vi "Test - With DRAM.vi"() -> ()   [LabVIEW 2020, in "Raster (FPGA).lvlib"]
uses:
  Raster (FPGA).lvlib
  Triangle.ctl
  Vertex.ctl
  Vector 3D.ctl
  UV.ctl
  <vilib>/rvi/Emulation/niFpgaGetClockAttributes.vi
  <vilib>/rvi/Emulation/niFpgaSctlEmulationGetInTimedLoop.vi
  <vilib>/rvi/Emulation/niFpgaEmulationReportErrorSimple.vi
  <vilib>/rvi/Emulation/niFpgaCriticalErrorInLSC.vi
  <vilib>/rvi/DataTransferAndStorage/Container/XNode/niFpgaContainer.xnode
  <vilib>/rvi/Memory/Memory_Emulation/niFpgaMemoryFastEmulationDramWriteAndRequestData.vi
  <vilib>/rvi/Memory/Memory_Emulation/niFpgaMemoryEmulationDramWriteAndRequestData.vi
  <vilib>/platform/TimedLoop/XDataNode/XDataNode.xnode
  <vilib>/Platform/TimedLoop/XDataNode/nitl_modes.ctl
  <vilib>/Platform/TimedLoop/XDataNode/XDNodeRunTimeDep.lvlib
  <vilib>/Platform/TimedLoop/XDataNode/wakeup.ctl
  <vilib>/Platform/TimedLoop/XDataNode/timing_clust.ctl
  <vilib>/rvi/interface/RandomDataEmulation/nirviRandomDataFpgaReadWriteTemplate.vi
  <vilib>/rvi/FIFO/Fifo_Resource/nirvififoEmulationRead.vi
  <vilib>/rvi/FIFO/Fifo_Resource/nirvififoEmulationWrite.vi
  <instrlib>/_niInstr/Basic Elements/v1/FPGA/niInstr Basic Elements v1 FPGA.lvlib
  <vilib>/rvi/Memory/Memory_Emulation/niFpgaMemoryEmulationDramRetrieveData.vi
panel:
  out "Element":cluster{"Address":i32, "Value":u32}
  out "To Host Timed Out? 2":bool
  in  "Send To Host 2":bool
  out "DRAM Read Address 2":u32
  out "Raster Loop Period [us]":u32
  in  "Raster Loop Wait [ticks]":u32=10000 caption="Count(uSec)"
  out "To DRAM Timed Out?":bool
  out "Raster Loop Index":i32
  in  "Triangle":T1={"Vertex 1"={"Position"={"x"=75.0, "y"=25.0, "z"=0.0}, "UV"={"u"=0.0, "v"=0.0}, "Colour"=12517256}, "Vertex 2"={"Position"={"x"=500.0, "y"=450.0, "z"=0.0}, "UV"={"u"=0.0, "v"=0.0}, "Colour"=12517256}, "Vertex 3"={"Position"={"x"=50.0, "y"=200.0, "z"=0.0}, "UV"={"u"=0.0, "v"=0.0}, "Colour"=12517256}, "Colour"=5308226} {"Vertex 3"."UV"."v" min=0 max=1 step=0.1; "Vertex 3"."UV"."u" min=0 max=1 step=0.1; "Vertex 2"."UV"."v" min=0 max=1 step=0.1; "Vertex 2"."UV"."u" min=0 max=1 step=0.1; "Vertex 1"."UV"."v" min=0 max=1 step=0.1; "Vertex 1"."UV"."u" min=0 max=1 step=0.1}
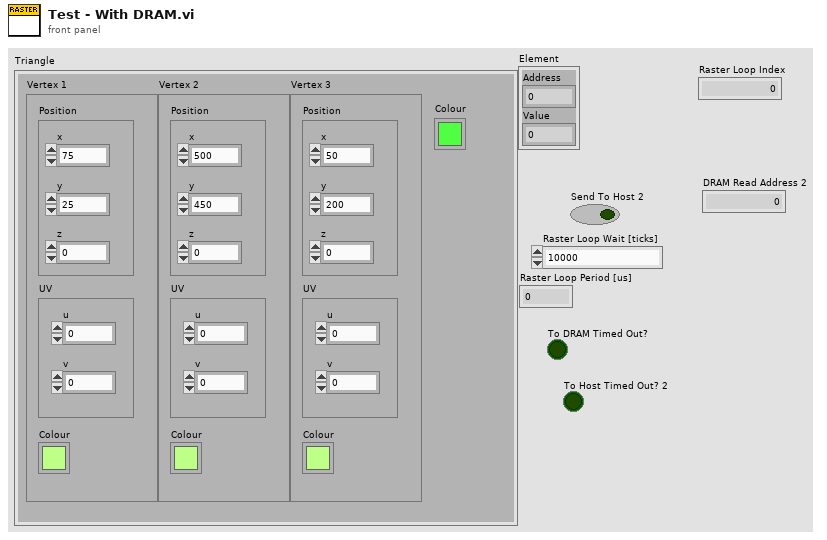
[diagram p1: front panel]
types:
  T1 = typedef "Raster (FPGA).lvlib/Triangle.ctl" = cluster{"Vertex 1":T2, "Vertex 2":T2, "Vertex 3":T2, "Colour":u32}
  T2 = typedef "Raster (FPGA).lvlib/Vertex.ctl" = cluster{"Position":T3, "UV":T4, "Colour":u32}
  T3 = typedef "Raster (FPGA).lvlib/Vector 3D.ctl" = cluster{"x":sgl, "y":sgl, "z":sgl}
  T4 = typedef "Raster (FPGA).lvlib/UV.ctl" = cluster{"u":sgl, "v":sgl}
  T5 = typedef "Raster (FPGA).lvlib/Triangle (Sorted).ctl" = cluster{"Top Vertex":T2, "Mid Vertex":T2, "Bottom Vertex":T2, "Colour":u32}
  T6 = typedef "Raster (FPGA).lvlib/Reciprocals.ctl" = cluster{"Bottom --> Top":sgl, "Bottom --> Middle":sgl, "Middle --> Top":sgl}
  T7 = typedef "Raster (FPGA).lvlib/Current Row.ctl" = cluster{"Start Column":sgl, "End Column":sgl}
  T8 = typedef "XDNodeRunTimeDep.lvlib/timing_clust.ctl" = cluster{"Expected End [f-1]":u64, "Actual End [f-1]":u64, "Finished Late? [f-1]":bool, "Expected End [i-1]":u64, "Actual End [i-1]":u64, "Finished Late? [i-1]":bool, "Expected Start [i]":u64, "Actual Start [i]":u64, "Expected Start [f]":u64, "Actual Start [f]":u64, "Source Name":string, "Structure Name":string, "Period":i64, "Deadline":i64, "Offset":i64, "Start":i64, "Priority":i32, "Timeout":i32, "Mode":T9, "Wakeup Reason":T10, "Error":errorcluster, "Source Type":string, "Secondary Source Type":string, "Global End Time":u64, "Global Start Time":u64, "Frame Duration":u64, "Iteration Duration":u64, "Assigned CPU":i32, "I/O Scan Engine Mode":u32}
  T9 = typedef "XDNodeRunTimeDep.lvlib/nitl_modes.ctl" = enum32{"No Change", "Process missed periods, maintain original phase", "Discard missed periods, maintain original phase", "Process missed periods, ignore original phase", "Discard missed periods, ignore original phase"}
  T10 = typedef "XDNodeRunTimeDep.lvlib/wakeup.ctl" = enum32{"Normal", "Aborted", "Asynchronous wakeup", "Timing source error", "Timed loop error", "Timeout"}
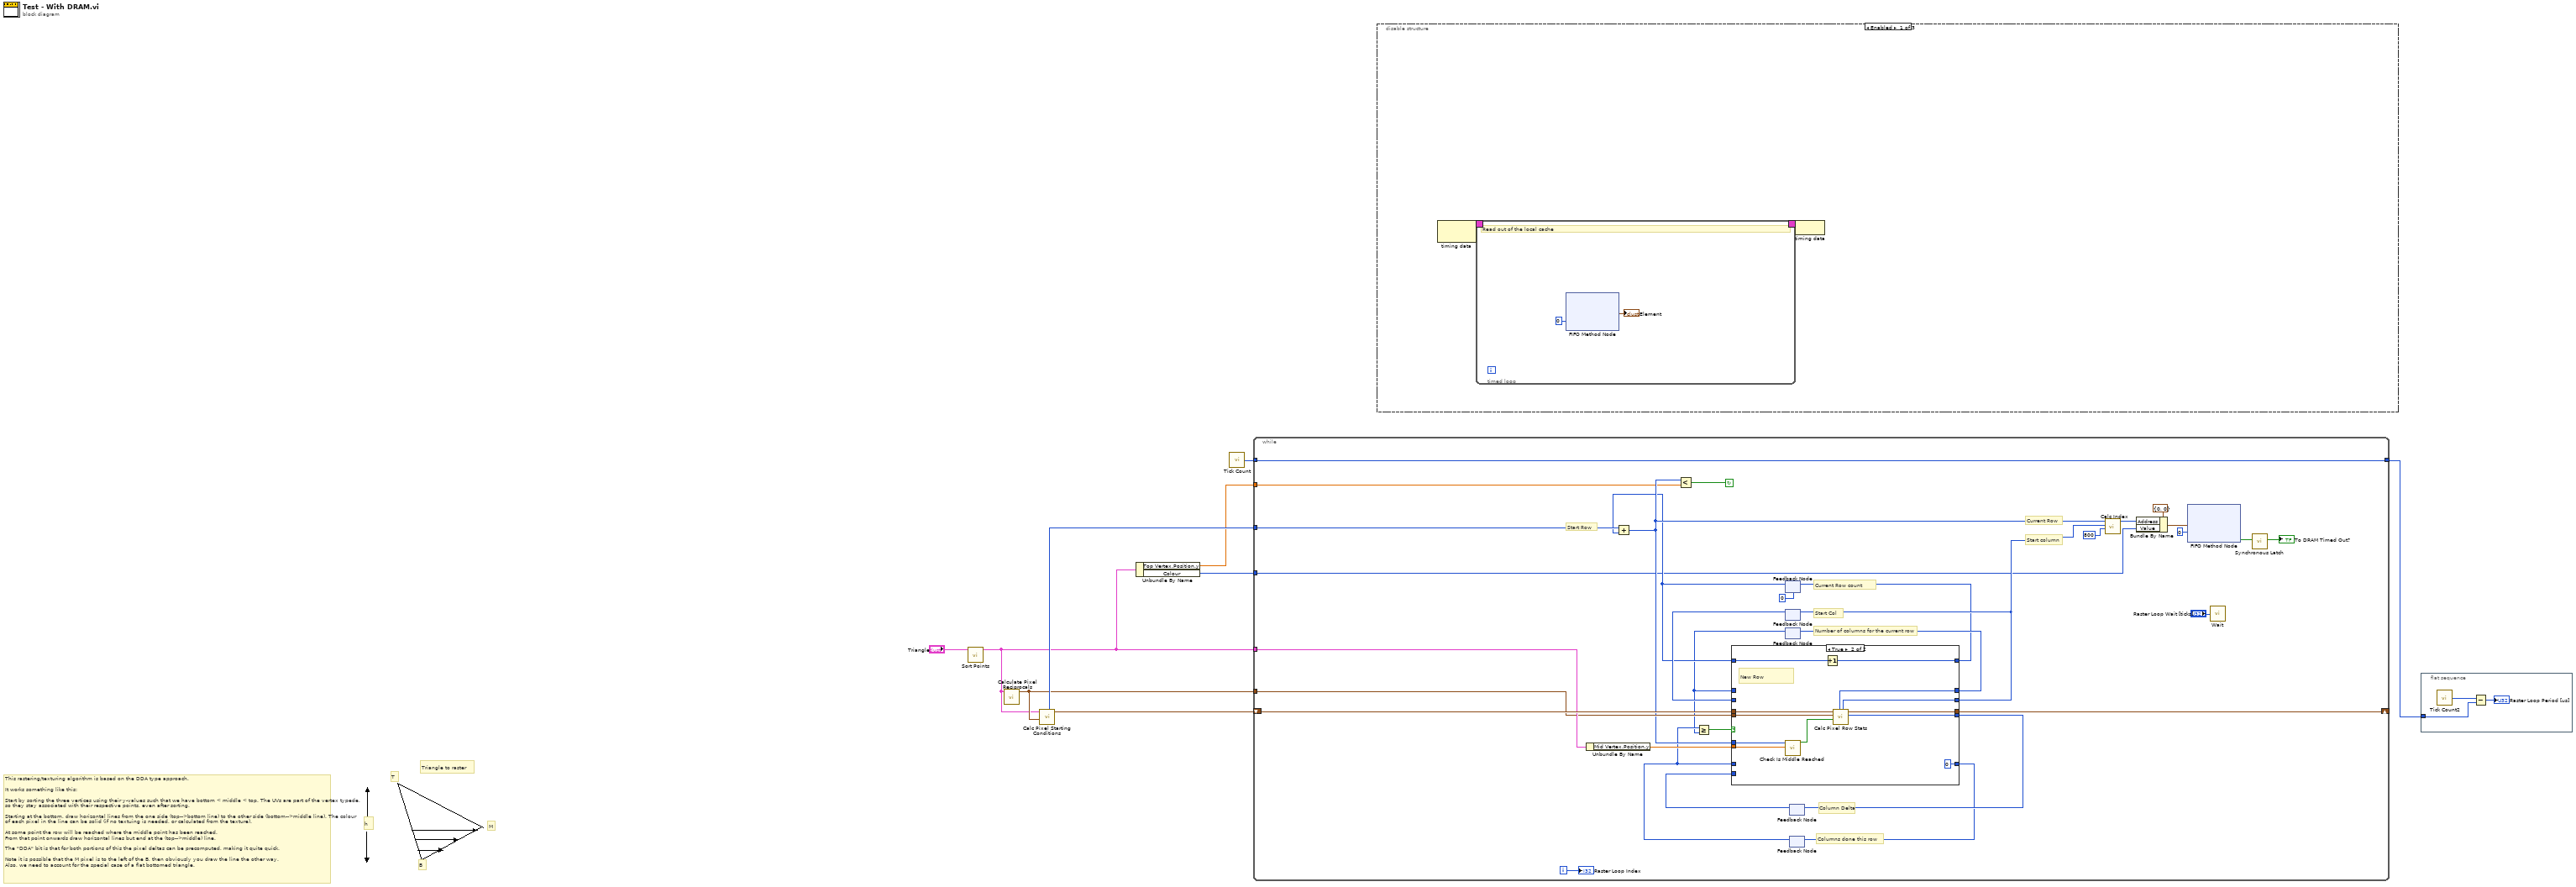
[diagram p0: block diagram]
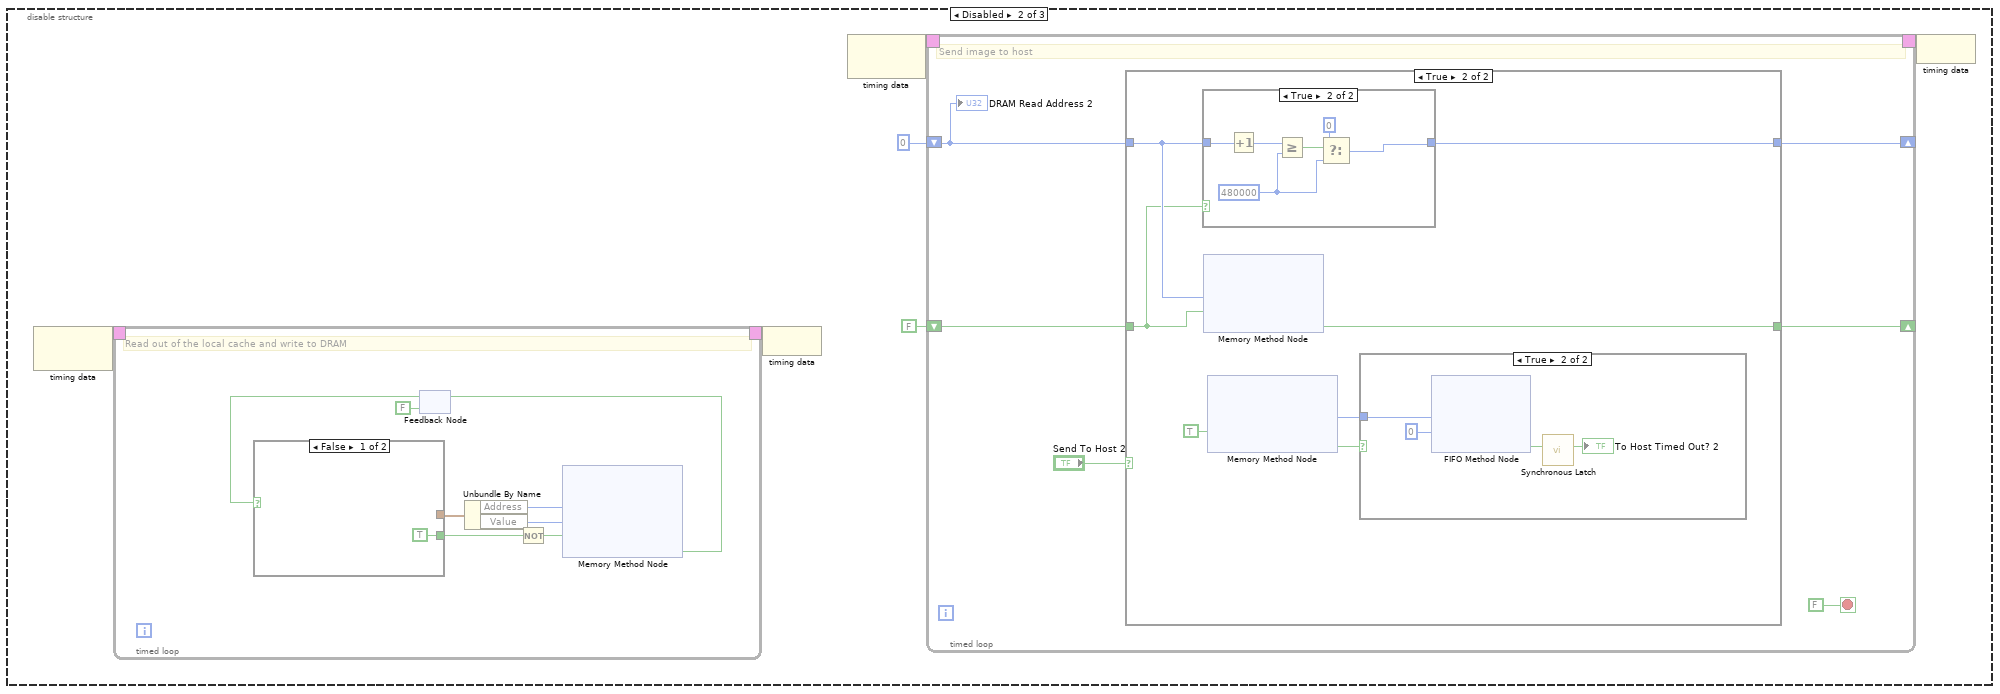
[diagram p2: hidden frame]
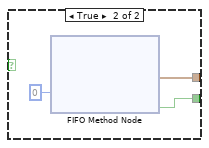
[diagram p6: hidden frame]
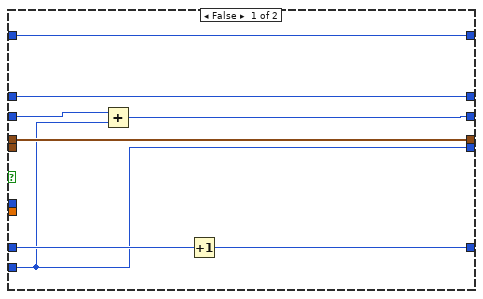
[diagram p8: hidden frame]
diagram:
  # "h"
  # "Triangle to raster"
  # "M"
  # "T"
  # "B"
  # "This rastering/texturing algorithm is based on the DDA type approach.\n\nIt works something like this:\n\nStart by sorting the three vertices using their y-values such that we have bottom < middle < top. The UVs are part of the vertex typede, so they stay associated with their respective points, even after sorting.\n\nStarting at the bottom, draw horizontal lines from the one side (top-->bottom line) to the other side (bottom-->middle line). The colour of each pixel in the line can be solid (if no textuing is needed, or calculated from the texture).\n\nAt some point the row will be reached where the middle point has been reached.\nFrom that point onwards draw horizontal lines but end at the (top-->middle) line.\n\nThe \"DDA\" bit is that for both portions of this the pixel deltas can be precomputed, making it quite quick.\n\nNote it is possible that the M pixel is to the left of the B, then obviously you draw the line the other way.\nAlso, we need to account for the special case of a flat bottomed triangle."
  n1 = call "Sort Points.vi"("Triangle"="Triangle") -> ("Sorted Triangle"=w4:T5)  [unwired: 10 in]
  n2 = call "Calculate Pixel Reciprocals.vi"("Sorted Triangle"=w4) -> ("Columns Pixels Per Row"=w6:T6)  [unwired: 10 in]
  n3 = call "Calc Pixel Starting Conditions.vi"("Reciprocals"=w6, "Sorted Vertices (V1 is top)"=w4) -> ("Start Row Columns"=w9:T7, "Start Row"=w8:i32)  [unwired: 8 in]
  n4 = Unbundle By Name(w4) -> ("Top Vertex.Position.y"=w3:sgl, "Colour"=w5:u32)
  n5 = call "Tick Count"() -> ("Tick Count(uSec)"=w2:u32)
  n6 = while {
    shift-right: [w39] -> _
    shift-left: w9 -> [w37]
    tunnel: w4 -> [w36]
    tunnel: w8 -> [w38]
    tunnel: w6 -> [w34]
    tunnel: w5 -> [w15]
    tunnel: w3 -> [w32]
    tunnel: w2 -> [w13]
    tunnel: [w13] -> w1
    i -> [w35]
    stop <- w40 continue-if-true
    # "Columns done this row"
    # "Column Delta"
    # "Current Row count"
    # "Start Col"
    # "Number of columns for the current row"
    # "Current Row"
    # "Start column"
    # "Start Row"
    n7 = Unbundle By Name(w36) -> ("Mid Vertex.Position.y"=w41:sgl)
    n8 = feedback #1(0) -> (w24:i32)
    n9 = Add(x=w38, y=w24) -> (x+y=w33:i32)
    n10 = Less?(x=w33, y=w32) -> (x < y?=w40:bool)
    n11 = feedback #2() -> (w29:i32)  [unwired: 1 in]
    n12 = feedback #3() -> (w21:i32)  [unwired: 1 in]
    n13 = feedback #4() -> (w27:i32)  [unwired: 1 in]
    n14 = feedback #5() -> (w22:i32)  [unwired: 1 in]
    n15 = Greater Or Equal?(x=w22, y=w21) -> (x >= y?=w20:bool)
    n16 = case shown="True" w20 {
      tunnel: w41 -> [_ w61]
      tunnel: [w48 w60] -> w39
      tunnel: w37 -> [w48 w59]
      tunnel: w34 -> [_ w58]
      tunnel: [w49 w57] -> w31
      tunnel: [w42 w55] -> w28
      tunnel: [w43 w54] -> w30
      tunnel: w33 -> [_ w53]
      tunnel: w21 -> [w49 _]
      tunnel: w29 -> [w44 _]
      tunnel: w27 -> [w42 _]
      tunnel: w24 -> [w47 w52]
      tunnel: [w47 w51] -> w25
      tunnel: [w45 0] -> w23
      tunnel: w22 -> [w46 _]
      frame False {
        n17 = Add(x=w44, y=w42) -> (x+y=w43:i32)
        n18 = Increment(x=w46) -> (x+1=w45:i32)
      }
      frame True {
        # "New Row"
        n19 = call "Check Is Middle Reached.vi"("Middle y"=w61, "Current Row"=w53) -> ("Reached Middle"=w56:bool)  [unwired: 9 in]
        n20 = Increment(x=w52) -> (x+1=w51:i32)
        n21 = call "Calc Pixel Row Stats.vi"("Reached Middle"=w56, "Reciprocals"=w58, "Current Row"=w59) -> ("Column Delta"=w55:i32, "Next Row"=w60:T7, "Start Col"=w54:i32, "Number Of Cols This Row"=w57:i32)  [unwired: 4 in, 1 out]
      }
    }
    n22 = feedback-in #1(w25) -> ()
    n23 = feedback-in #2(w30) -> ()
    n24 = feedback-in #3(w31) -> ()
    n25 = feedback-in #4(w28) -> ()
    n26 = feedback-in #5(w23) -> ()
    n27 = call "Calc Index.vi"("Cols Per Row"=800, "Col"=w30, "Row"=w33) -> ("Index"=w16:i32)  [unwired: 8 in]
    n28 = Bundle By Name(cluster=cluster{"Address":i32, "Value":u32} {"Address"=0, "Value"=0} ("Element"), "Address"=w16, "Value"=w15) -> (w17:cluster{"Address":i32, "Value":u32})
    n29 = xnode ("FIFO Method Node")("Element"=w17, "Timeout"=0) -> ("Timed Out?"=w10:bool)  [unwired: 1 in, 1 out]
    n30 = call "Wait"("Count(Ticks)"="Raster Loop Wait [ticks]") -> ()  [unwired: 1 out]
    n31 = call <instrlib>:"Synchronous Latch.vi"("set"=w10) -> ("out"=→"To DRAM Timed Out?":bool)  [unwired: 10 in]
    "Raster Loop Index" <- w35
  }
  n32 = disable-structure shown="Enabled" {
    frame Enabled {
      n33 = node-c288() -> (w63:T8)  [unwired: 1 in]
      n34 = timed-loop {
        timing: w63 -> [_]
        timing-out: [_] -> w62
        stop <- FALSE stop-if-true
        # "Read out of the local cache"
        n35 = xnode ("FIFO Method Node")("Timeout"=0) -> ("Element"=→"Element":cluster{"Address":i32, "Value":u32})  [unwired: 1 in, 2 out]
      }
      n36 = node-c288(w62) -> ()
    }
    frame Disabled {
      n37 = node-c288() -> (w76:T8)  [unwired: 1 in]
      n38 = timed-loop {
        timing: w76 -> [_]
        timing-out: [_] -> w75
        stop <- FALSE stop-if-true
        # "Read out of the local cache and write to DRAM"
        n39 = feedback #6(FALSE ("Ready for Input")) -> (w108:bool)
        n40 = case shown="False" w108 {
          tunnel: [TRUE ("Timed Out?") w119] -> w114
          tunnel: [_ w117] -> w112
          frame False {
          }
          frame True {
            n41 = xnode ("FIFO Method Node")("Timeout"=0) -> ("Element"=w117:cluster{"Address":i32, "Value":u32}, "Timed Out?"=w119:bool)  [unwired: 1 in, 1 out]
          }
        }
        n42 = Unbundle By Name(w112) -> ("Address"=w111:i32, "Value"=w110:u32)
        n43 = Not(x=w114) -> (.not. x?=w113:bool)
        n44 = xnode ("Memory Method Node")("Address"=w111, "Data"=w110, "Input Valid"=w113) -> ("Ready for Input"=w109:bool)  [unwired: 1 in, 1 out]
        n45 = feedback-in #6(w109) -> ()
      }
      n46 = node-c288(w75) -> ()
      n47 = node-c288() -> (w74:T8)  [unwired: 1 in]
      n48 = timed-loop {
        timing: w74 -> [_]
        timing-out: [_] -> w73
        shift-right: [w78] -> _
        shift-left: u32 0 ("t") -> [w77]
        shift-right: [w80] -> _
        shift-left: FALSE ("Ready for Input") -> [w79]
        stop <- FALSE stop-if-true
        # "Send image to host"
        n49 = case shown="True" "Send To Host 2" {
          tunnel: w77 -> [w84 w88]
          tunnel: [w83 w89] -> w80
          tunnel: w79 -> [w83 w85]
          tunnel: [w84 w87] -> w78
          frame False {
          }
          frame True {
            n50 = case shown="True" w85 {
              tunnel: w88 -> [w92 w95]
              tunnel: [w92 w94] -> w87
              frame False {
              }
              frame True {
                w93 = u32 480000
                n51 = Increment(x=w95) -> (x+1=w98:u32)
                n52 = Greater Or Equal?(x=w98, y=w93) -> (x >= y?=w96:bool)
                n53 = Select(t=u32 0, s=w96, f=w93) -> (s? t:f=w94:u32)
              }
            }
            n54 = xnode ("Memory Method Node")("Address"=w88, "Input Valid"=w85) -> ("Ready for Input"=w89:bool)  [unwired: 1 in, 1 out]
            n55 = xnode ("Memory Method Node")("Ready for Output"=TRUE) -> ("Data"=w90:i16, "Output Valid"=w91:bool)  [unwired: 1 in, 1 out]
            n56 = case shown="True" w91 {
              tunnel: w90 -> [_ w102]
              frame False {
              }
              frame True {
                n57 = xnode ("FIFO Method Node")("Element"=w102, "Timeout"=0) -> ("Timed Out?"=w99:bool)  [unwired: 1 in, 1 out]
                n58 = call <instrlib>:"Synchronous Latch.vi"("set"=w99) -> ("out"=→"To Host Timed Out? 2":bool)  [unwired: 10 in]
              }
            }
          }
        }
        "DRAM Read Address 2" <- w77
      }
      n59 = node-c288(w73) -> ()
    }
    frame Disabled {
    }
  }
  n60 = flat-sequence {
    tunnel: w1 -> [w125]
    frame #0 {
      n61 = call "Tick Count2"() -> ("Tick Count(uSec)"=w126:u32)
      n62 = Subtract(x=w126, y=w125) -> (x-y=→"Raster Loop Period [us]":u32)
    }
  }
